vi "Логи_приемника.vi"() -> ()   [LabVIEW 2013]
panel:
  in  "Tab Control":enum32{"Входные сигналы приемника", "Стик"}(tab)
  out "XY Graph 2":cluster{dbl[], dbl[]}[](graph)
  out "XY Graph 3":cluster{dbl[], dbl[]}[](graph)
  out "Array 2":i16[](array[numeric])
  out "Array":i16[](array[numeric])
  out "ID параметров":u8[](array[numeric])
  out "Длина заголовка":i32
  out "Заголовок":string
  out "Количество параметров":u8
  out "size (in bytes)":i64
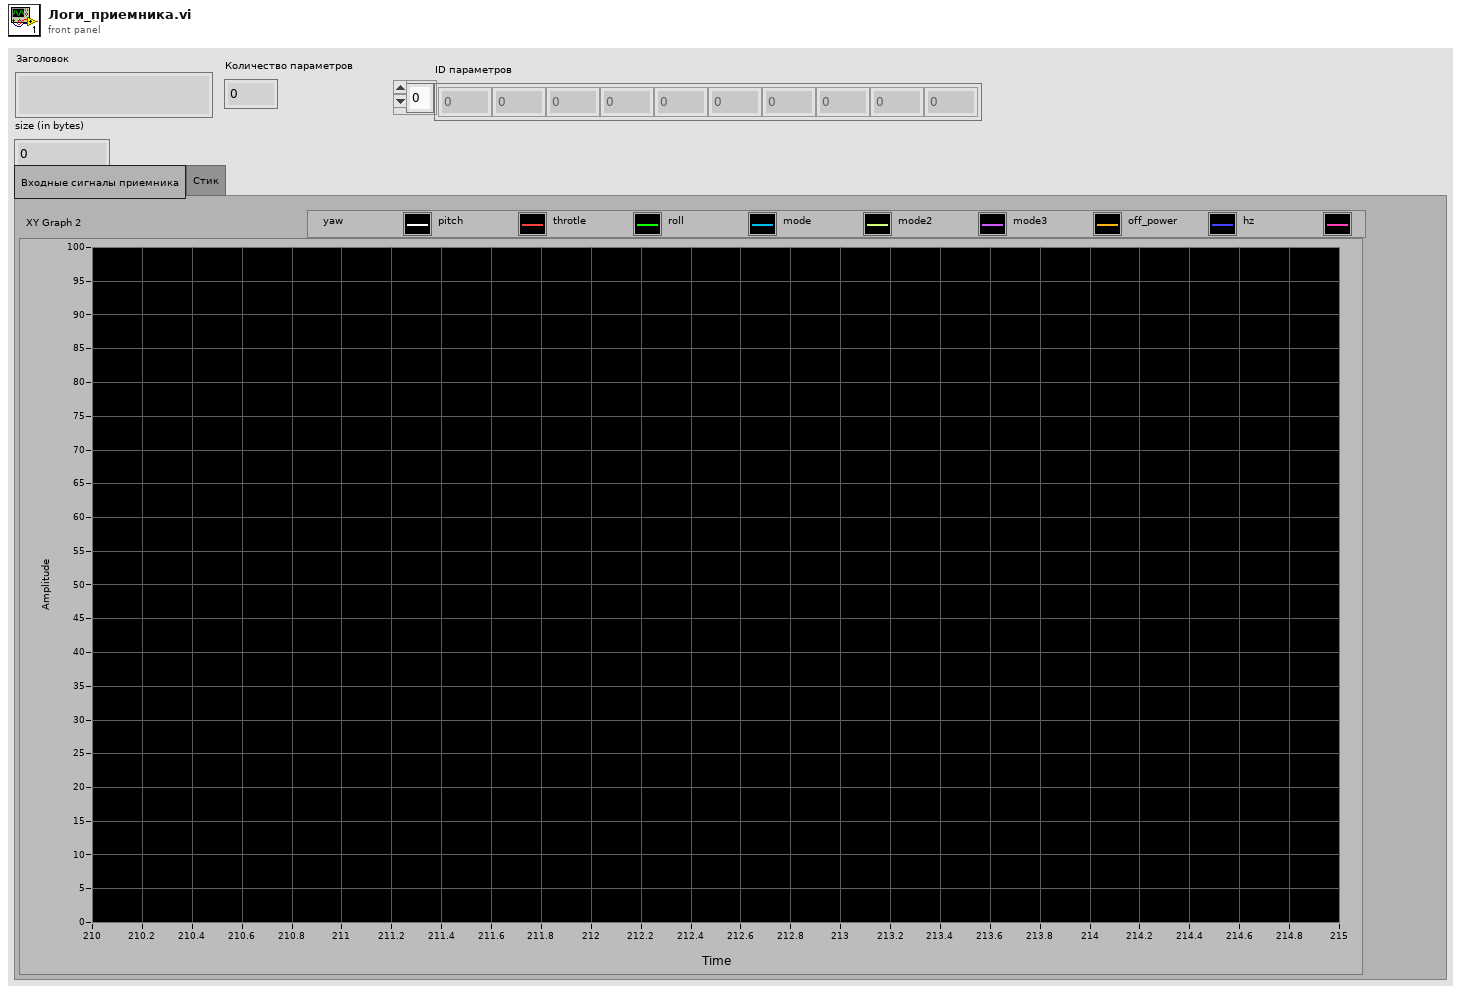
[diagram p1: front panel]
types:
  T1 = enum16{"open", "replace", "create", "open or create", "replace or create", "replace or create with confirmation"}
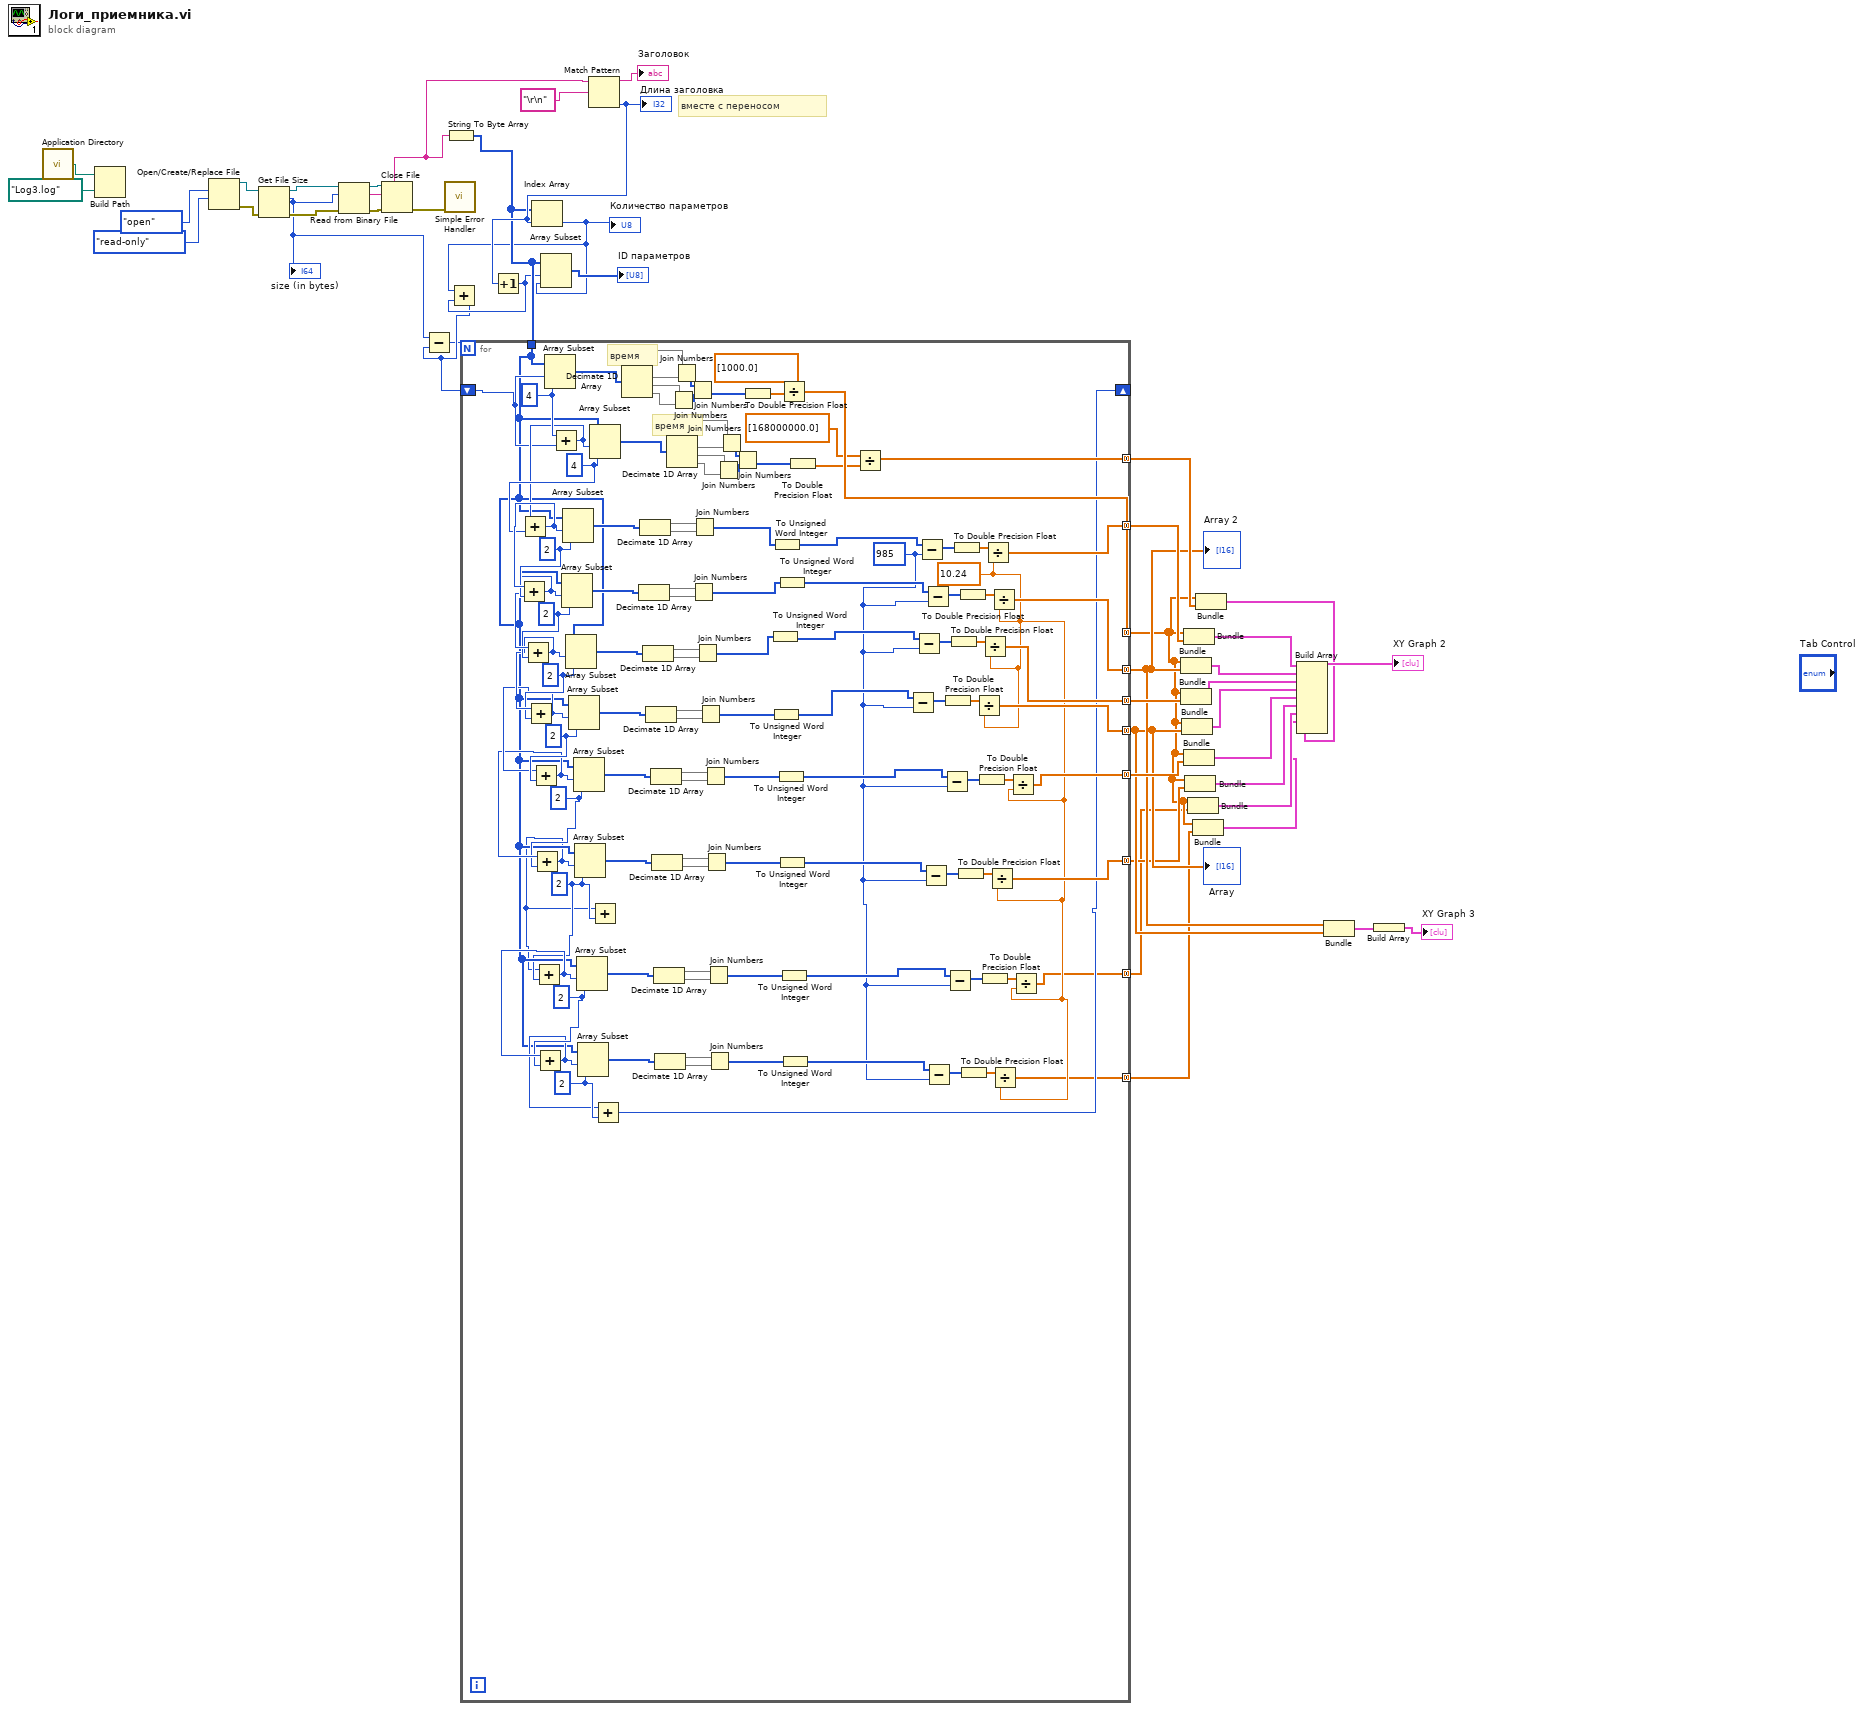
[diagram p0: block diagram]
diagram:
  # "вместе с переносом"
  n1 = call <vilib>:"Application Directory.vi"() -> ("Application Directory"=w41:path)
  n2 = Build Path(base path=w41, name or relative path=path "Log3.log" ("default name")) -> ()  [unwired: 1 out]
  n3 = Open/Create/Replace File(operation (0:open)=T1."open", access (0:read/write)=enum16{"read/write", "read-only", "write-only"}."read-only") -> (refnum out=w38:refnum<file>, error out=w36:errorcluster)  [unwired: 4 in, 1 out]
  n4 = Get File Size(file=w38, error in=w36) -> (refnum out=w37:refnum<file>, size (in bytes)=w28:i64, 0:w35:errorcluster)
  "size (in bytes)" <- w28
  n5 = Read from Binary File(8:w35, 10:w28, 11:w37) -> (0:w39:errorcluster, 2:w34:string, 3:w40:refnum<file>)  [unwired: 3 in, 1 out]
  n6 = Close File(refnum=w40, error in=w39) -> (error out=w44:errorcluster)  [unwired: 1 out]
  n7 = call <vilib>:"Simple Error Handler.vi"("error in (no error)"=w44) -> ()  [unwired: 4 in, 5 out]
  n8 = String To Byte Array(string=w34) -> (unsigned byte array=w29:u8[])
  n9 = Match Pattern(string=w34, regular expression="\r\n" ("format string")) -> (before substring=→"Заголовок":string, offset past match=w31:i32)  [unwired: 1 in, 2 out]
  "Длина заголовка" <- w31
  n10 = Increment(x=w31) -> (x+1=w26:i32)
  n11 = Index Array(array=w29, index=w31) -> (element=w27:u8)
  "Количество параметров" <- w27
  n12 = Add(x=w27, y=w26) -> (x+y=w25:i32)
  n13 = Subtract(x=w28, y=w25) -> (x-y=w24:i64)
  n14 = for {
    N: w24 -> [_]
    tunnel: w29 -> [w51]
    shift-right: [w49] -> _
    shift-left: w25 -> [w101]
    tunnel: [w126] -> w5 mode=concatenating
    tunnel: [w73] -> w22 mode=concatenating
    tunnel: [w71] -> w10 mode=concatenating
    tunnel: [w75] -> w21 mode=concatenating
    tunnel: [w78] -> w9 mode=concatenating
    tunnel: [w79] -> w16 mode=concatenating
    tunnel: [w102] -> w15 mode=concatenating
    tunnel: [w91] -> w8 mode=concatenating
    tunnel: [w46] -> w4 mode=concatenating
    tunnel: [w45] -> w6 mode=concatenating
    w62 = 2 ("length")
    w60 = 2 ("length")
    w47 = 10.24 ("y")
    w52 = u16 985 ("y")
    w50 = 2 ("length")
    w106 = 4 ("length")
    w95 = 2 ("length")
    w117 = 2 ("length")
    w127 = 2 ("length")
    w129 = 2 ("length")
    w131 = 2 ("length")
    w107 = 4 ("length")
    # "время"
    # "время"
    n15 = Array Subset(array=w51, index=w101, length=w107) -> (w148:u8[])
    n16 = Add(x=w107, y=w101) -> (x+y=w105:i32)
    n17 = Add(x=w105, y=w106) -> (x+y=w132:i32)
    n18 = Add(x=w132, y=w131) -> (x+y=w130:i32)
    n19 = Add(x=w130, y=w129) -> (x+y=w128:i32)
    n20 = Add(x=w128, y=w127) -> (x+y=w116:i32)
    n21 = Add(x=w116, y=w117) -> (x+y=w96:i32)
    n22 = Add(x=w96, y=w95) -> (x+y=w48:i32)
    n23 = Add(x=w48, y=w50) -> (x+y=w61:i32)
    n24 = Add(x=w61, y=w60) -> (x+y=w59:i32)
    n25 = Array Subset(array=w51, index=w130, length=w129) -> (w139:u8[])
    n26 = Array Subset(array=w51, index=w132, length=w131) -> (w142:u8[])
    n27 = Array Subset(array=w51, index=w128, length=w127) -> (w136:u8[])
    n28 = Array Subset(array=w51, index=w116, length=w117) -> (w133:u8[])
    n29 = Array Subset(array=w51, index=w96, length=w95) -> (w119:u8[])
    n30 = Array Subset(array=w51, index=w48, length=w50) -> (w98:u8[])
    n31 = Array Subset(array=w51, index=w61, length=w60) -> (w68:u8[])
    n32 = Array Subset(array=w51, index=w59, length=w62) -> (w64:u8[])
    n33 = Array Subset(array=w51, index=w105, length=w106) -> (w109:u8[])
    n34 = Add(x=w48, y=w50) -> ()  [unwired: 1 out]
    n35 = Add(x=w59, y=w62) -> (x+y=w49:i32)
    n36 = Decimate 1D Array(w148) -> (w150:u8[], w151:u8[], w152:u8[], w153:u8[])
    n37 = Decimate 1D Array(w139) -> (w140:u8[], w141:u8[])
    n38 = Decimate 1D Array(w142) -> (w143:u8[], w144:u8[])
    n39 = Decimate 1D Array(w136) -> (w137:u8[], w138:u8[])
    n40 = Decimate 1D Array(w133) -> (w134:u8[], w135:u8[])
    n41 = Decimate 1D Array(w119) -> (w120:u8[], w121:u8[])
    n42 = Decimate 1D Array(w98) -> (w99:u8[], w100:u8[])
    n43 = Decimate 1D Array(w68) -> (w69:u8[], w70:u8[])
    n44 = Decimate 1D Array(w64) -> (w65:u8[], w66:u8[])
    n45 = Decimate 1D Array(w109) -> (w111:u8[], w112:u8[], w113:u8[], w114:u8[])
    n46 = Join Numbers(hi=w152, lo=w153) -> ((hi.lo)=w149:u16[])
    n47 = Join Numbers(hi=w150, lo=w151) -> ((hi.lo)=w154:u16[])
    n48 = Join Numbers(hi=w154, lo=w149) -> ((hi.lo)=w145:u32[])
    n49 = Join Numbers(hi=w140, lo=w141) -> ((hi.lo)=w122:u16[])
    n50 = Join Numbers(hi=w143, lo=w144) -> ((hi.lo)=w125:u16[])
    n51 = Join Numbers(hi=w137, lo=w138) -> ((hi.lo)=w123:u16[])
    n52 = Join Numbers(hi=w134, lo=w135) -> ((hi.lo)=w124:u16[])
    n53 = Join Numbers(hi=w120, lo=w121) -> ((hi.lo)=w118:u16[])
    n54 = Join Numbers(hi=w99, lo=w100) -> ((hi.lo)=w97:u16[])
    n55 = Join Numbers(hi=w69, lo=w70) -> ((hi.lo)=w67:u16[])
    n56 = Join Numbers(hi=w65, lo=w66) -> ((hi.lo)=w63:u16[])
    n57 = Join Numbers(hi=w113, lo=w114) -> ((hi.lo)=w110:u16[])
    n58 = Join Numbers(hi=w111, lo=w112) -> ((hi.lo)=w115:u16[])
    n59 = Join Numbers(hi=w115, lo=w110) -> ((hi.lo)=w108:u32[])
    n60 = To Double Precision Float(number=w145) -> (double precision float=w147:dbl[])
    n61 = To Unsigned Word Integer(number=w123) -> (unsigned 16bit integer=w76:u16[])
    n62 = To Unsigned Word Integer(number=w124) -> (unsigned 16bit integer=w77:u16[])
    n63 = To Unsigned Word Integer(number=w125) -> (unsigned 16bit integer=w74:u16[])
    n64 = To Unsigned Word Integer(number=w118) -> (unsigned 16bit integer=w80:u16[])
    n65 = To Unsigned Word Integer(number=w122) -> (unsigned 16bit integer=w72:u16[])
    n66 = To Unsigned Word Integer(number=w97) -> (unsigned 16bit integer=w92:u16[])
    n67 = Divide(x=w147, y=dbl[] [1000.0]) -> (x/y=w126:dbl[])
    n68 = To Unsigned Word Integer(number=w67) -> (unsigned 16bit integer=w53:u16[])
    n69 = To Unsigned Word Integer(number=w63) -> (unsigned 16bit integer=w56:u16[])
    n70 = To Double Precision Float(number=w108) -> (double precision float=w104:dbl[])
    n71 = Divide(x=dbl[] [168000000.0] ("y"), y=w104) -> (x/y=w102:dbl[])
    n72 = Subtract(x=w77, y=w52) -> (x-y=w84:u16[])
    n73 = Subtract(x=w76, y=w52) -> (x-y=w86:u16[])
    n74 = Subtract(x=w74, y=w52) -> (x-y=w90:u16[])
    n75 = Subtract(x=w92, y=w52) -> (x-y=w94:u16[])
    n76 = Subtract(x=w72, y=w52) -> (x-y=w88:u16[])
    n77 = Subtract(x=w56, y=w52) -> (x-y=w58:u16[])
    n78 = Subtract(x=w80, y=w52) -> (x-y=w82:u16[])
    n79 = To Double Precision Float(number=w84) -> (double precision float=w83:dbl[])
    n80 = Subtract(x=w53, y=w52) -> (x-y=w55:u16[])
    n81 = To Double Precision Float(number=w86) -> (double precision float=w85:dbl[])
    n82 = To Double Precision Float(number=w90) -> (double precision float=w89:dbl[])
    n83 = To Double Precision Float(number=w94) -> (double precision float=w93:dbl[])
    n84 = To Double Precision Float(number=w88) -> (double precision float=w87:dbl[])
    n85 = To Double Precision Float(number=w58) -> (double precision float=w57:dbl[])
    n86 = Divide(x=w83, y=w47) -> (x/y=w78:dbl[])
    n87 = To Double Precision Float(number=w82) -> (double precision float=w81:dbl[])
    n88 = Divide(x=w85, y=w47) -> (x/y=w75:dbl[])
    n89 = To Double Precision Float(number=w55) -> (double precision float=w54:dbl[])
    n90 = Divide(x=w89, y=w47) -> (x/y=w73:dbl[])
    n91 = Divide(x=w93, y=w47) -> (x/y=w91:dbl[])
    n92 = Divide(x=w87, y=w47) -> (x/y=w71:dbl[])
    n93 = Divide(x=w57, y=w47) -> (x/y=w45:dbl[])
    n94 = Divide(x=w81, y=w47) -> (x/y=w79:dbl[])
    n95 = Divide(x=w54, y=w47) -> (x/y=w46:dbl[])
  }
  "Array" <- w9
  "Array 2" <- w10
  n96 = Array Subset(array=w29, index=w26, length=w27) -> (→"ID параметров":u8[])
  n97 = Bundle(w5, w10) -> (w14:cluster{dbl[], dbl[]})  [unwired: 1 in]
  n98 = Bundle(w5, w21) -> (w19:cluster{dbl[], dbl[]})  [unwired: 1 in]
  n99 = Bundle(w5, w9) -> (w11:cluster{dbl[], dbl[]})  [unwired: 1 in]
  n100 = Bundle(w5, w22) -> (w20:cluster{dbl[], dbl[]})  [unwired: 1 in]
  n101 = Bundle(w5, w16) -> (w17:cluster{dbl[], dbl[]})  [unwired: 1 in]
  n102 = Bundle(w5, w8) -> (w7:cluster{dbl[], dbl[]})  [unwired: 1 in]
  n103 = Bundle(w5, w4) -> (w3:cluster{dbl[], dbl[]})  [unwired: 1 in]
  n104 = Bundle(w5, w6) -> (w2:cluster{dbl[], dbl[]})  [unwired: 1 in]
  n105 = Bundle(w5, w15) -> (w1:cluster{dbl[], dbl[]})  [unwired: 1 in]
  n106 = Build Array(w20, w14, w19, w11, w17, w7, w3, w2, w1) -> (→"XY Graph 2":cluster{dbl[], dbl[]}[])
  n107 = Bundle(w10, w9) -> (w13:cluster{dbl[], dbl[]})  [unwired: 1 in]
  n108 = Build Array(w13) -> (→"XY Graph 3":cluster{dbl[], dbl[]}[])
